vi "set_AOTF_OnOffMod_forAll.vi"(8 "VISA Error In":errorcluster, 11 "on/off/mod":string) -> (0 "VISA Error Out":errorcluster)   [LabVIEW 2015]
panel:
  in  "Array 2":string[](array[string])
  in  "Array":string[](array[string])
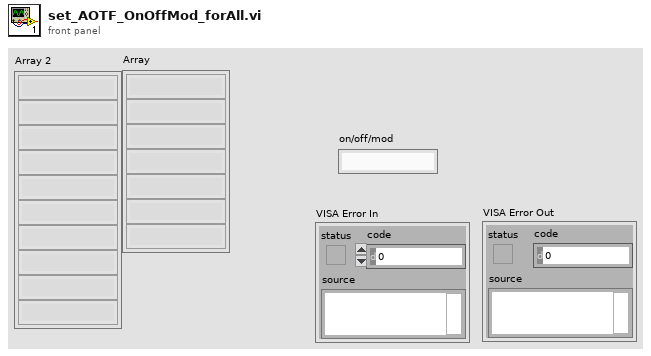
[diagram p1: front panel]
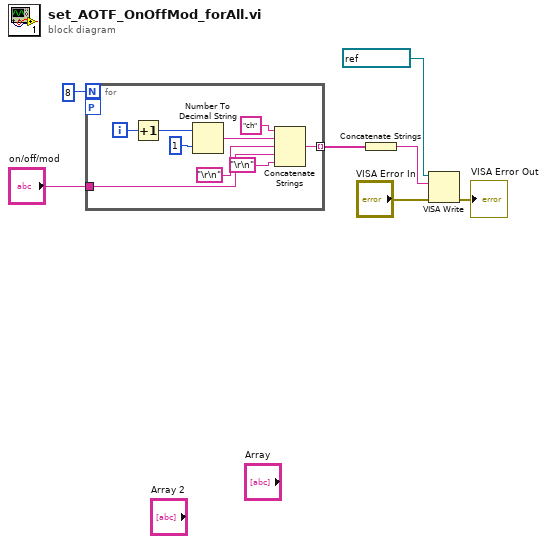
[diagram p0: block diagram]
diagram:
  n1 = for {
    N: 8 -> [_]
    workers-P: _ -> [_]
    tunnel: "on/off/mod" -> [w11]
    tunnel: [w10] -> w4 mode=indexing
    i -> [w9]
    n2 = Increment(x=w9) -> (x+1=w8:i32)
    n3 = Number To Decimal String(number=w8, width (-)=i16 1) -> (decimal integer string=w13:string)
    n4 = Concatenate Strings("ch", w13, "\r\n", w11, "\r\n") -> (w10:string)
  }
  n5 = Concatenate Strings(w4) -> (w3:string)
  n6 = VISA Write(VISA resource name=refnum<visa-resource-name> "COM13" ("COM channel"), write buffer=w3, error in (no error)="VISA Error In") -> (error out=→"VISA Error Out":errorcluster)  [unwired: 2 out]
